vi "ARGB Colour to U32 Pixel Value.vi"(1 "ARGB Colour":T1={"Alpha"=255, "RGB"=0}) -> (0 "U32 Colour":u32 format="%08x")   [LabVIEW 2020, in "g_ar_toolkit.image.lvlib"]
uses:
  g_ar_toolkit.image.lvlib
  ARGB Colour.ctl
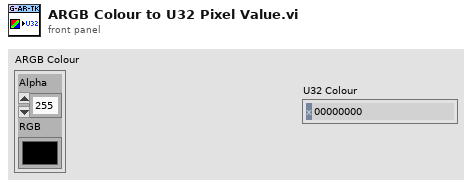
[diagram p1: front panel]
types:
  T1 = typedef "g_ar_toolkit.image.lvlib/ARGB Colour.ctl" = cluster{"Alpha":u8, "RGB":u32}
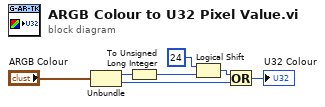
[diagram p0: block diagram]
diagram:
  n1 = Unbundle("ARGB Colour") -> ("Alpha"=w6:u8, "RGB"=w2:u32)
  n2 = To Unsigned Long Integer(number=w6) -> (unsigned 32bit integer=w5:u32)
  n3 = Logical Shift(y=i16 24, x=w5) -> (x << y=w3:u32)
  n4 = Or(x=w3, y=w2) -> (x .or. y?=→"U32 Colour":u32)
